vi "monochromatorCommandSetShutter.vi"(8 "error in":errorcluster, 10 "shutter":bool, 11 "monochromator":refnum<k24>) -> (0 "error out":errorcluster, 3 "monochromator":refnum<k24>)   [LabVIEW 2009]
doc: "SET shutter \nFALSE = Close shutter\nTRUE = Open shutter"
uses:
  C:/Users/anderson.chen/Desktop/Software Development/Cornerstone Series API (LV9)/Cornerstone DLL/Cornerstone.dll
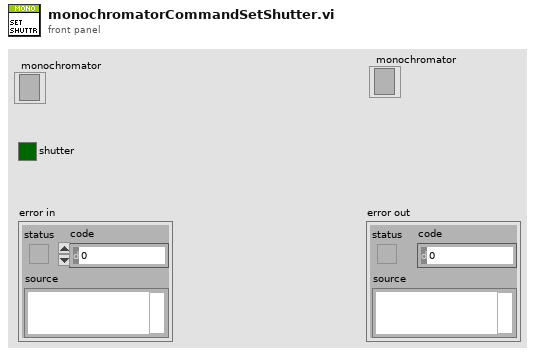
[diagram p1: front panel]
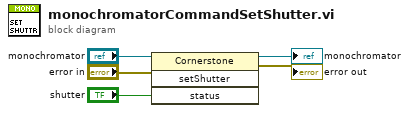
[diagram p0: block diagram]
diagram:
  n1 = invoke class="Cornerstone" method="setShutter"(reference="monochromator", error in="error in", "status"="shutter") -> (reference out=→"monochromator":refnum<k24>, error out=→"error out":errorcluster)  [unwired: 1 in, 2 out]
